vi "DAQ_tester.vi"() -> ()   [LabVIEW 2010]
uses:
  <vilib>/Utility/error.llb/DialogType.ctl
  <vilib>/ULx/Create Channel.llb/ULx Create Channel (AI-Voltage-Basic).vi
  <vilib>/ULx/Timing.llb/ULx Timing (Sample Clock).vi
  <vilib>/ULx/Create Channel.llb/ULx Create Channel (CO-Pulse Generation-Frequency).vi
  <vilib>/ULx/Write.llb/ULx Write (Analog 1D DBL 1Chan NSamp).vi
  <vilib>/ULx/Read.llb/ULx Read (Analog 1D DBL 1Chan NSamp).vi
panel:
  out "Waveform Chart":dbl[](graph)
  in  "AI":refnum<k21>
  out "number of samples written per channel":u32
  in  "Boolean":bool
  in  "Output":refnum<k21>
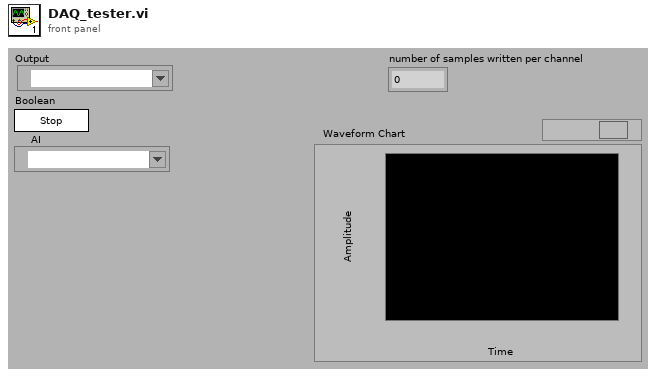
[diagram p1: front panel]
types:
  T1 = typedef "DialogType.ctl" = u16
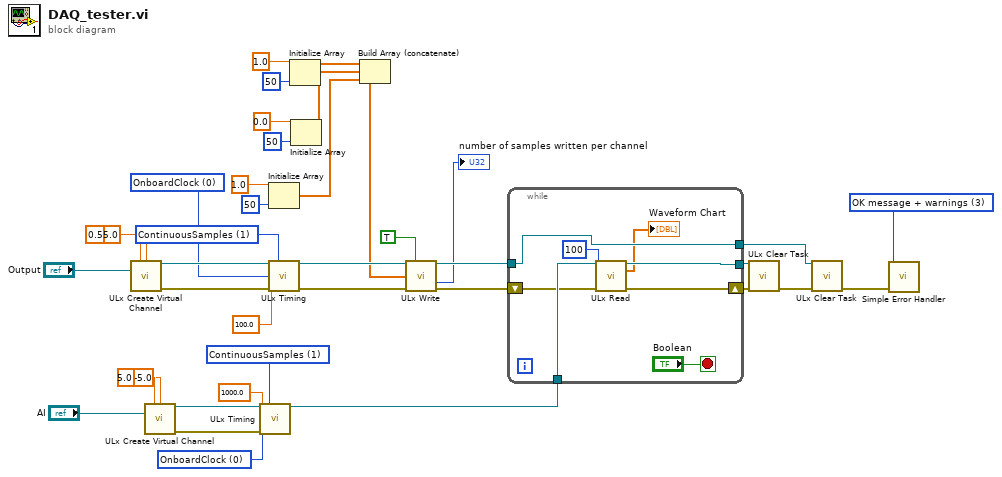
[diagram p0: block diagram]
diagram:
  w9 = 1 items=["FiniteSamples", "ContinuousSamples"] ("sample mode")
  w10 = 0 items=["OnboardClock", "ExternalClock", "NoClock"] ("clock source")
  w21 = T1 3 items=["no dialog", "OK message", "continue or stop message", "OK message + warnings", "continue/stop + warnings"] ("type of dialog (OK msg:1)")
  w34 = 1 items=["FiniteSamples", "ContinuousSamples"] ("sample mode")
  w36 = 0 items=["OnboardClock", "ExternalClock", "NoClock"] ("clock source")
  n1 = call-poly <vilib>:"ULx Create Virtual Channel.vi"("frequency"=5.0, "duty cycle"=0.5, "counters"="Output") -> ("task out"=w38:refnum<k24>, "error out"=w37:errorcluster)  [unwired: 11 in]
  n2 = call-poly <vilib>:"ULx Create Virtual Channel.vi"("maximum value"=5.0, "minimum value"=-5.0, "physical channels"="AI") -> ("task out"=w12:refnum<k24>, "error out"=w13:errorcluster)  [unwired: 11 in]
  n3 = call-poly <vilib>:"ULx Timing.vi"("task in"=w12, "sample mode"=w9, "rate"=1000.0, "clock source"=w10, "error in"=w13) -> ("task out"=w8:refnum<k24>)  [unwired: 9 in, 1 out]
  n4 = Initialize Array(1.0 ("element"), 50 ("dimension size")) -> (w18:dbl[])
  n5 = call-poly <vilib>:"ULx Timing.vi"("task in"=w38, "sample mode"=w34, "rate"=100.0, "clock source"=w36, "error in"=w37) -> ("task out"=w33:refnum<k24>, "error out"=w32:errorcluster)  [unwired: 9 in]
  n6 = Initialize Array(1.0 ("element"), 50 ("dimension size")) -> (w24:dbl[])
  n7 = Initialize Array(0.0 ("element"), 50 ("dimension size")) -> (w23:dbl[])
  n8 = Build Array (concatenate)(w24, w23, w18) -> (w17:dbl[])
  n9 = call-poly <vilib>:"ULx Write.vi"("task in"=w33, "auto start"=TRUE, "data"=w17, "error in"=w32) -> ("task out"=w30:refnum<k24>, "number of samples written per channel"=→"number of samples written per channel":u32, "error out"=w29:errorcluster)  [unwired: 9 in]
  n10 = while {
    tunnel: w30 -> [w41]
    shift-right: [w44] -> w6
    shift-left: w29 -> [w45]
    tunnel: w8 -> [w46]
    tunnel: [w42] -> w7
    tunnel: [w41] -> w4
    stop <- "Boolean" stop-if-true
    n11 = call-poly <vilib>:"ULx Read.vi"("task in"=w46, "number of samples per channel"=100, "error in"=w45) -> ("task out"=w42:refnum<k24>, "data"=→"Waveform Chart":dbl[], "error out"=w44:errorcluster)  [unwired: 10 in]
  }
  n12 = call <vilib>:"ULx Clear Task.vi"("task in"=w7, "error in"=w6) -> ("error out"=w5:errorcluster)  [unwired: 13 in]
  n13 = call <vilib>:"ULx Clear Task.vi"("task in"=w4, "error in"=w5) -> ("error out"=w3:errorcluster)  [unwired: 13 in]
  n14 = call <vilib>:"Simple Error Handler.vi"("type of dialog (OK msg:1)"=w21, "error in (no error)"=w3) -> ()  [unwired: 3 in, 5 out]
